vi "2468 Manipulator Constants.vi"() -> ()   [LabVIEW 2020]
panel:
  in  "2468 Intake Presets":T1(array[cluster])=[{"Preset Name"="Intake", "Cone"=0.9, "Cube"=-0.5}, {"Preset Name"="Outtake/Score", "Cone"=-0.5, "Cube"=0.6}, {"Preset Name"="Idle", "Cone"=0.075, "Cube"=-0.05}]
  in  "2468 Manipulator Config":T2={"Safe Wrist Position"=0.35, "Margin of Error"={"Safety Wrist Margin"=0.03, "Cascade Margin"=2.0, "Final Wrist Margin"=0.03}, "grid-dy"=[{"Griddy Preset"="idle", "cascade pos"=0.0, "wrist pos"=0.25}, {"Griddy Preset"="intake cone", "cascade pos"=0.0, "wrist pos"=0.62}, {"Griddy Preset"="intake cube", "cascade pos"=0.0, "wrist pos"=0.54}, {"Griddy Preset"="score low cone", "cascade pos"=0.0, "wrist pos"=0.5}, {"Griddy Preset"="score low cube", "cascade pos"=0.0, "wrist pos"=0.25}, {"Griddy Preset"="score mid cone", "cascade pos"=21.4, "wrist pos"=0.75}, {"Griddy Preset"="score mid cube", "cascade pos"=8.7, "wrist pos"=0.3}, {"Griddy Preset"="score high cone", "cascade pos"=21.4, "wrist pos"=0.57}, {"Griddy Preset"="score high cube", "cascade pos"=19.4, "wrist pos"=0.4}]}
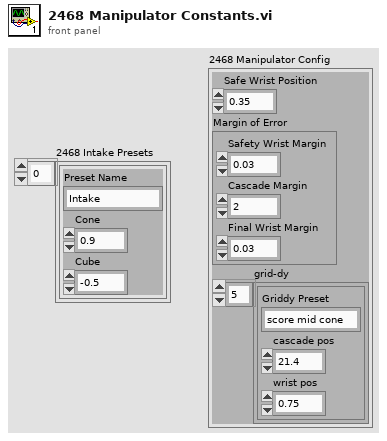
[diagram p1: front panel]
types:
  T1 = cluster{"Preset Name":string, "Cone":dbl, "Cube":dbl}[]
  T2 = cluster{"Safe Wrist Position":dbl, "Margin of Error":cluster{"Safety Wrist Margin":dbl, "Cascade Margin":dbl, "Final Wrist Margin":dbl}, "grid-dy":cluster{"Griddy Preset":string, "cascade pos":dbl, "wrist pos":dbl}[]}
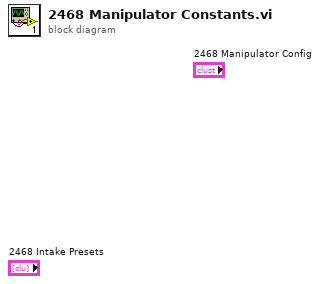
[diagram p0: block diagram]
diagram:
